vi "ScanparametersToFPGA.vi"(8 "error in":errorcluster, 9 "Parameters In":T3={"fastRoundPts"=32, "slowRoundPts"=8, "fastWaveType"=enum."Rounded", "slowWaveType"=enum."Triangle", "fastWavePts"=1024, "slowWavePts"=1024, "outputRateHz"=800000, "yOffset"=0.0, "xOffset"=0.0, "scanSizeSlow"=0.5, "scanSizeFast"=0.5, "rotation"=0.0, "timePerLine"=0.01, "numLines"=256, "pointsPerLine"=512, "scanEnable"=FALSE, "slowMoveWavePts"=1024, "slowMoveAccelPts"=128, "moveSpeedSec"=0.2, "singleDirectionScan"=FALSE} {"yOffset" min=0.0 max=1.0 format="%#_6p"; "xOffset" min=0.0 max=1.0 format="%#_6p"; "scanSizeSlow" min=0.0 max=1.0 format="%#_6p"; "scanSizeFast" min=0.0 max=1.0 format="%#_6p"; "timePerLine" min=0.001 max=100.0 format="%#_6p"; "outputRateHz" format="%.0p"}, 11 "FPGAIn":T1) -> (0 "error out":errorcluster, 1 "Parameters In to Send back":T3={"fastRoundPts"=32, "slowRoundPts"=8, "fastWaveType"=enum."Rounded", "slowWaveType"=enum."Triangle", "fastWavePts"=1024, "slowWavePts"=1024, "outputRateHz"=800000, "yOffset"=0.0, "xOffset"=0.0, "scanSizeSlow"=0.5, "scanSizeFast"=0.5, "rotation"=0.0, "timePerLine"=0.01, "numLines"=256, "pointsPerLine"=512, "scanEnable"=FALSE, "slowMoveWavePts"=1024, "slowMoveAccelPts"=128, "moveSpeedSec"=0.2, "singleDirectionScan"=FALSE} {"yOffset" min=0.0 max=1.0 format="%#_6p"; "xOffset" min=0.0 max=1.0 format="%#_6p"; "scanSizeSlow" min=0.0 max=1.0 format="%#_6p"; "scanSizeFast" min=0.0 max=1.0 format="%#_6p"; "timePerLine" min=0.001 max=100.0 format="%#_6p"; "outputRateHz" format="%.0p"}, 2 "Real Param":T2, 3 "FPGAOut":T1, 4 "timePerLineNew":dbl)   [LabVIEW 2016]
uses:
  FGV/ScanParametersAllTypeDef.ctl
  controls/ScanWaveform.ctl
  controls/FPGAVIreferenceTypeDefScanEngine.ctl
  controls/Enum.ctl
  <vilib>/Analysis/coordinate.llb/2D Cartesian Coordinate Rotation (Scalar).vi
  <vilib>/rvi/errors/niLvFpgaAdjustHostInterfaceError.vi
  <vilib>/Utility/error.llb/Error Cluster From Error Code.vi
  <vilib>/rvi/interface/nirviReadWriteControl/nirviReadWriteControl.xnode
  FPGA Bitfiles/qnmController797_usbRIO_controllerFPGAmu.lvbitx
  <vilib>/Analysis/NI_AALPro.lvlib
  NiFpgaLv.dll
panel:
  out "ioClock":dbl
  out "frequencyDec":i32
  out "realOutputFrequency":dbl
  # "scanWaveFormCtl"
  # "slowMoveParameters"
  # "scanCtl"
  # "ioParams"
  # "scanWaveFormCtl"
  # "slowMoveParameters"
  # "scanCtl"
  # "ioParams"
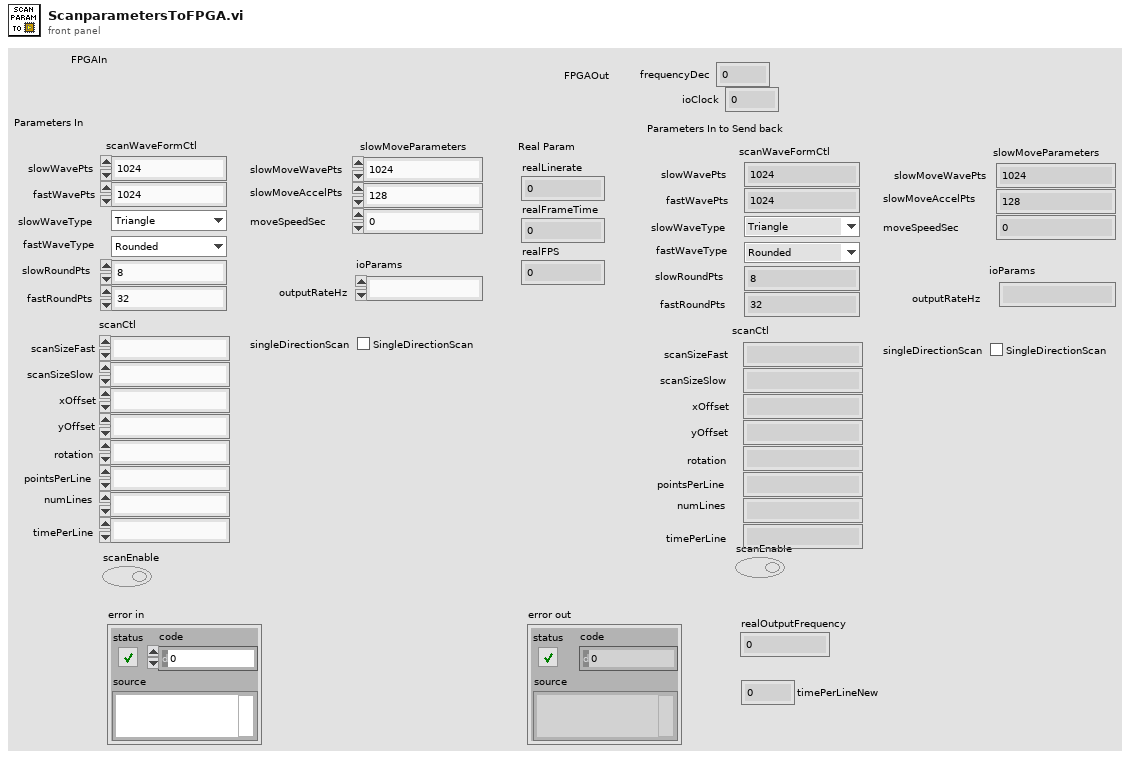
[diagram p1: front panel]
types:
  T1 = typedef "FPGAVIreferenceTypeDefScanEngine.ctl" = refnum<k20>
  T2 = cluster{"realFPS":dbl, "realLinerate":dbl, "realFrameTime":dbl}
  T3 = typedef "ScanParametersAllTypeDef.ctl" = cluster{"fastRoundPts":u16, "slowRoundPts":u16, "fastWaveType":T4, "slowWaveType":T4, "fastWavePts":u16, "slowWavePts":u16, "outputRateHz":u32, "yOffset":dbl, "xOffset":dbl, "scanSizeSlow":dbl, "scanSizeFast":dbl, "rotation":dbl, "timePerLine":dbl, "numLines":u16, "pointsPerLine":u32, "scanEnable":bool, "slowMoveWavePts":u16, "slowMoveAccelPts":u16, "moveSpeedSec":dbl, "singleDirectionScan":bool}
  T4 = typedef "ScanWaveform.ctl" = enum16{"Sine", "Triangle", "Rounded"}
  T5 = typedef "Enum.ctl" = enum16{"Init", "Read", "Write"}
  T6 = cluster{"a":fxp<+/-,18,2>, "b":fxp<+/-,18,2>, "c":fxp<+/-,18,2>, "d":fxp<+/-,18,2>}
  T7 = cluster{"fastScanSize":fxp<+,17,1>, "slowScanSize":fxp<+,17,1>, "invertSlowAxis":bool}
  T8 = cluster{"outputRate":u16, "fastDecFactor":u16, "outWaveSizeFast":u16, "pplUpsampling":u16, "numLines":u16, "se.p.fastInvDec":fxp<+,22,0>, "se.p.slowUpStep":fxp<+,28,0>, "se.p.outWaveSizeSlow":u16, "blankingMax":u32, "se.p.fastBlanking":cluster{"startFwd":u32, "endFwd":u32, "startBwd":u32, "endBwd":u32, "disableBlanking":bool, "useCoarseCounter":bool}}
  T9 = cluster{"startFwd":u32, "endFwd":u32, "startBwd":u32, "endBwd":u32, "disableBlanking":bool, "useCoarseCounter":bool}
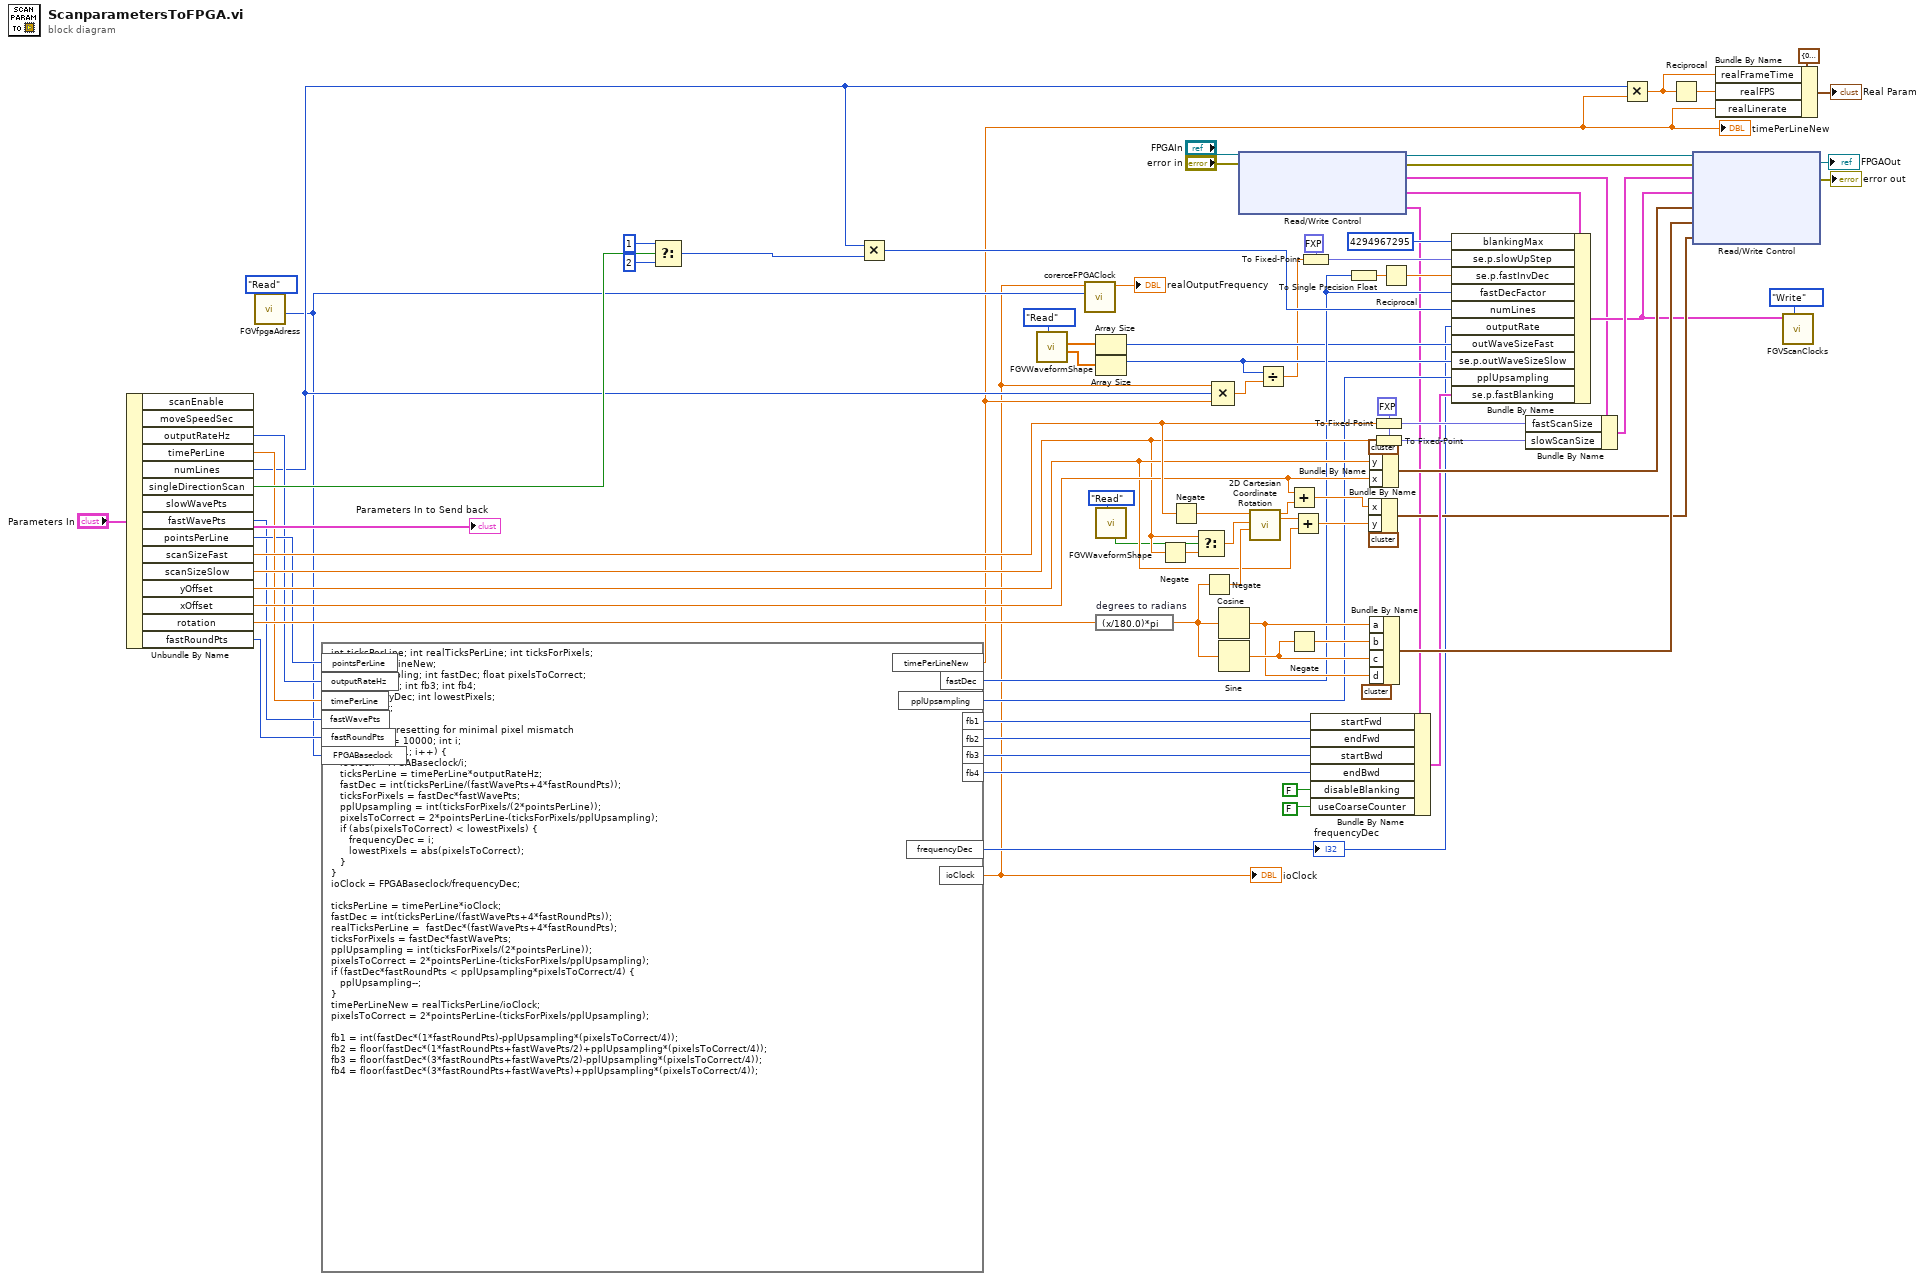
[diagram p0: block diagram]
diagram:
  w45 = fxp<+,17,1> 0.0 ("fastScanSize")
  n1 = Unbundle By Name("Parameters In") -> ("outputRateHz"=w20:u32, "timePerLine"=w44:dbl, "numLines"=w16:u16, "singleDirectionScan"=w73:bool, "fastWavePts"=w42:u16, "pointsPerLine"=w43:u32, "scanSizeFast"=w82:dbl, "scanSizeSlow"=w50:dbl, "yOffset"=w51:dbl, "xOffset"=w53:dbl, "rotation"=w74:dbl, "fastRoundPts"=w41:u16)  [unwired: 3 out]
  n2 = call "FGVfpgaAdress.vi"("Enum"=Enum."Read") -> ("baseClockOut"=w15:u32)  [unwired: 5 in, 5 out]
  n3 = formula code="int ticksPerLine; int realTicksPerLine; int ticksForPixels;\nfloat timePerLineNew;\nint pplUpsampling; int fastDec; float pixelsToCorrect; \nint fb1; int fb2; int fb3; int fb4;\nint frequencyDec; int lowestPixels;\nfloat ioClock;\n\n// frequency presetting for minimal pixel mismatch\nlowestPixels = 10000; int i;\nfor (i=40; i < 81; i++) {\n   ioClock = FPGABaseclock/i;\n   ticksPerLine = timePerLine*outputRateHz;\n   fastDec = int(ticksPerLine/(fastWavePts+4*fastRoundPts));\n   ticksForPixels = fastDec*fastWavePts;\n   pplUpsampling = int(ticksForPixels/(2*pointsPerLine));\n   pixelsToCorrect = 2*pointsPerLine-(ticksForPixels/pplUpsampling);\n   if (abs(pixelsToCorrect) < lowestPixels) {\n      frequencyDec = i;\n      lowestPixels = abs(pixelsToCorrect);\n   }\n}\nioClock = FPGABaseclock/frequencyDec;\n\nticksPerLine = timePerLine*ioClock;\nfastDec = int(ticksPerLine/(fastWavePts+4*fastRoundPts));\nrealTicksPerLine =  fastDec*(fastWavePts+4*fastRoundPts);\nticksForPixels = fastDec*fastWavePts;\npplUpsampling = int(ticksForPixels/(2*pointsPerLine));\npixelsToCorrect = 2*pointsPerLine-(ticksForPixels/pplUpsampling);\nif (fastDec*fastRoundPts < pplUpsampling*pixelsToCorrect/4) {\n   pplUpsampling--;\n}\ntimePerLineNew = realTicksPerLine/ioClock;\npixelsToCorrect = 2*pointsPerLine-(ticksForPixels/pplUpsampling);\n\nfb1 = int(fastDec*(1*fastRoundPts)-pplUpsampling*(pixelsToCorrect/4));\nfb2 = floor(fastDec*(1*fastRoundPts+fastWavePts/2)+pplUpsampling*(pixelsToCorrect/4));\nfb3 = floor(fastDec*(3*fastRoundPts+fastWavePts/2)-pplUpsampling*(pixelsToCorrect/4));\nfb4 = floor(fastDec*(3*fastRoundPts+fastWavePts)+pplUpsampling*(pixelsToCorrect/4));"("pointsPerLine"=w43, "outputRateHz"=w20, "timePerLine"=w44, "fastWavePts"=w42, "fastRoundPts"=w41, "FPGABaseclock"=w15) -> ("timePerLineNew"=w2:dbl, "pplUpsampling"=w31:i32, "fastDec"=w34:i32, "fb1"=w40:i32, "fb2"=w39:i32, "fb3"=w38:i32, "fb4"=w37:i32, "frequencyDec"=w3:i32, "ioClock"=w1:dbl)
  "timePerLineNew" <- w2
  "frequencyDec" <- w3
  "ioClock" <- w1
  n4 = Select(t=u16 1, s=w73, f=u16 2 ("x")) -> (s? t:f=w17:u16)
  n5 = Multiply(x=w16, y=w17) -> (x*y=w64:u16)
  n6 = call "FGVWaveformShape.vi"("Enum"=Enum."Read") -> ("Waveform Shape Slow Out"=w67:dbl[], "Waveform Shape Fast Out"=w71:dbl[])  [unwired: 6 in, 3 out]
  n7 = call "corerceFPGAClock.vi"("baseClock"=w15, "requestedFrequency"=w1) -> ("realFrequency"=→"realOutputFrequency":dbl)  [unwired: 7 in, 2 out]
  n8 = Array Size(array=w71) -> (size(s)=w24:i32)
  n9 = Array Size(array=w67) -> (size(s)=w23:i32)
  n10 = call "FGVWaveformShape.vi"("Enum"=Enum."Read") -> ("Framing up? (down: f) out"=w48:bool)  [unwired: 6 in, 4 out]
  n11 = expression code="(x/180.0)*pi" "degrees to radians"(w74) -> (w52:dbl)
  n12 = Negate(x=w50) -> (-x=w62:dbl)
  n13 = Negate(x=w82) -> (-x=w60:dbl)
  n14 = Select(t=w50, s=w48, f=w62) -> (s? t:f=w56:dbl)
  n15 = Negate(x=w52) -> (-x=w54:dbl)
  n16 = Compound Arithmetic op=MULTIPLY(w1, w16, w2) -> (w22:dbl)
  n17 = Cosine(x=w52) -> (cos(x)=w75:dbl)
  n18 = Sine(x=w52) -> (sin(x)=w76:dbl)
  n19 = xnode "Read/Write Control"("FPGA VI Reference In"="FPGAIn", "error in"="error in") -> ("FPGA VI Reference Out"=w6:T1, "error out"=w9:errorcluster, "se.p.scanSize"=w13:T7, "se.p.clocks"=w12:T8, "se.p.clocks.se.p.fastBlanking"=w14:T9)
  n20 = call-poly <vilib>:"2D Cartesian Coordinate Rotation.vi"("theta"=w54, "y"=w56, "x"=w60) -> ("y out"=w57:dbl, "x out"=w61:dbl)  [unwired: 6 in, 1 out]
  n21 = Divide(x=w23, y=w22) -> (x/y=w21:dbl)
  n22 = Add(x=w53, y=w61) -> (x+y=w59:dbl)
  n23 = Negate(x=w76) -> (-x=w77:dbl)
  n24 = Add(x=w57, y=w51) -> (x+y=w58:dbl)
  n25 = To Fixed-Point(fixed-point type=fxp<+,28,0> 0.0 ("se.p.slowUpStep"), number=w21) -> (fixed-point=w28:fxp<+,28,0>)
  n26 = Bundle By Name(cluster=w14, "startFwd"=w40, "endFwd"=w39, "startBwd"=w38, "endBwd"=w37, "disableBlanking"=FALSE, "useCoarseCounter"=FALSE ("useFineCounter")) -> (w32:T9)
  n27 = To Single Precision Float(number=w34) -> (single precision float=w26:sgl)
  n28 = Bundle By Name(cluster=cluster{"x":fxp<+/-,16,1>, "y":fxp<+/-,16,1>} {"x"=0.0, "y"=0.0} ("moveToPoint"), "x"=w59, "y"=w58) -> (w29:cluster{"x":fxp<+/-,16,1>, "y":fxp<+/-,16,1>})
  n29 = Bundle By Name(cluster=cluster{"x":fxp<+/-,16,1>, "y":fxp<+/-,16,1>} {"x"=0.0, "y"=0.0} ("scanOffset"), "y"=w51, "x"=w53) -> (w66:cluster{"x":fxp<+/-,16,1>, "y":fxp<+/-,16,1>})
  n30 = Bundle By Name(cluster=T6 {"a"=0.0, "b"=0.0, "c"=0.0, "d"=0.0} ("outputMatrix"), "a"=w75, "b"=w77, "c"=w76, "d"=w75) -> (w65:T6)
  n31 = To Fixed-Point(fixed-point type=w45, number=w82) -> (fixed-point=w47:fxp<+,17,1>)
  n32 = To Fixed-Point(fixed-point type=w45, number=w50) -> (fixed-point=w46:fxp<+,17,1>)
  n33 = Reciprocal(x=w26) -> (1/x=w30:sgl)
  n34 = Bundle By Name(cluster=w12, "blankingMax"=u32 4294967295, "se.p.slowUpStep"=w28, "se.p.fastInvDec"=w30, "fastDecFactor"=w34, "numLines"=w64, "outputRate"=w3, "outWaveSizeFast"=w24, "se.p.outWaveSizeSlow"=w23, "pplUpsampling"=w31, "se.p.fastBlanking"=w32) -> (w25:T8)
  n35 = Bundle By Name(cluster=w13, "fastScanSize"=w47, "slowScanSize"=w46) -> (w63:T7)
  n36 = Multiply(x=w16, y=w2) -> (x*y=w18:dbl)
  n37 = Reciprocal(x=w18) -> (1/x=w68:dbl)
  n38 = xnode "Read/Write Control"("FPGA VI Reference In"=w6, "error in"=w9, "se.p.scanSize"=w63, "se.p.clocks"=w25, "se.p.scanOffsets"=w66, "se.p.transformMatrix"=w65, "se.mot.p.target"=w29) -> ("FPGA VI Reference Out"=→"FPGAOut":T1, "error out"=→"error out":errorcluster)
  n39 = Bundle By Name(cluster=T2 {"realFPS"=0.0, "realLinerate"=0.0, "realFrameTime"=0.0} ("Real Param"), "realFrameTime"=w18, "realFPS"=w68, "realLinerate"=w2) -> (→"Real Param":T2)
  n40 = call "FGVScanClocks.vi"("Enum"=Enum."Write", "scanClocksInput"=w25) -> ()  [unwired: 6 in, 2 out]
  "Parameters In to Send back" <- "Parameters In"
